vi "Stop_Exit.vi"(8 "error in (no error)":errorcluster, 10 "error in":errorcluster, 11 "STOP button":bool) -> (0 "error out":errorcluster, 3 "Exit While":bool)   [LabVIEW 2023]
doc: "This VI is just to keep the code clean and compact it ends the while loop when stop button is pressed or if an error occurs"
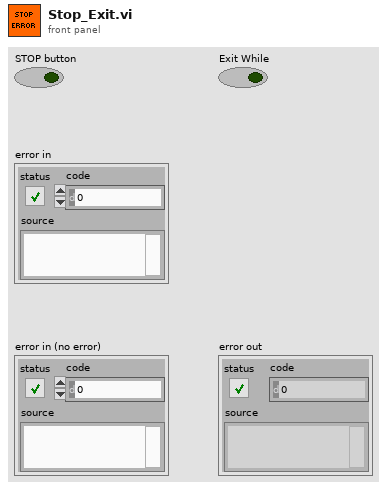
[diagram p1: front panel]
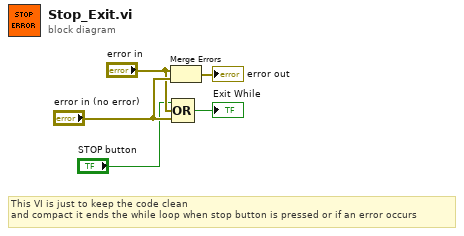
[diagram p0: block diagram]
diagram:
  # "This VI is just to keep the code clean \nand compact it ends the while loop when stop button is pressed or if an error occurs"
  n1 = Merge Errors("error in", "error in (no error)") -> (→"error out":errorcluster)
  n2 = Compound Arithmetic op=OR("STOP button", "error in", "error in (no error)") -> (→"Exit While":bool)
